vi "GlobalVariables.vi"() -> ()   [LabVIEW 2015]
panel:
  in  "Cursor1":T1
  in  "Cursor0":T1
  out "可识别数据类型":string="*.can;*.txt;*.asc;*.csv;*.trc;*.blf"
  in  "BinlogDLLPath":path
  in  "ConfigIniPath":path
  in  "YFormatsCopy":T2={"Ylimits"={"Upbound"=1.0, "Downbound"=0.0}, "ParentScaleID"=-1, "LabelTitle"=""}
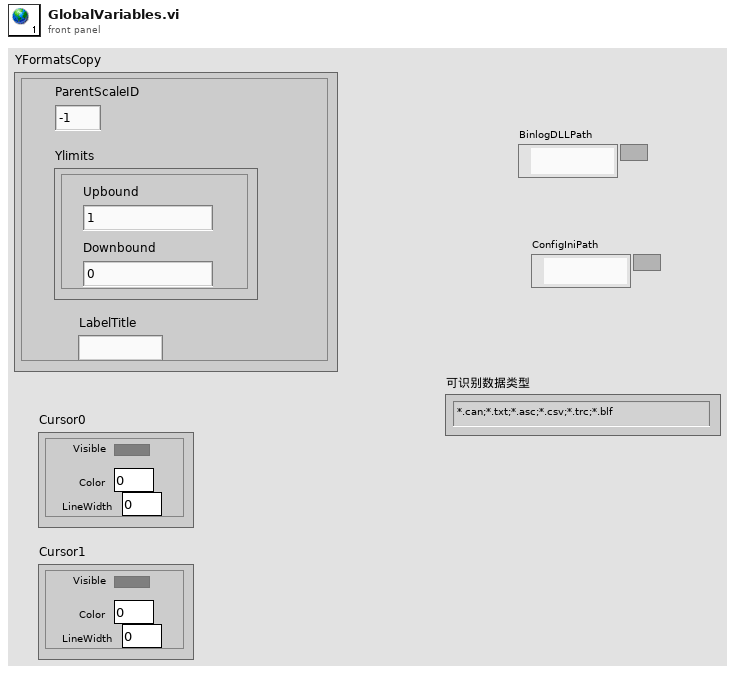
[diagram p1: front panel]
types:
  T1 = cluster{"Visible":bool, "Color":u32, "LineWidth":u8}
  T2 = cluster{"Ylimits":cluster{"Upbound":dbl, "Downbound":dbl}, "ParentScaleID":i32, "LabelTitle":string}
diagram:
